vi "SVI_SendSerialCommand.vi"(8 "error in (no error)":errorcluster, 9 "DAC Voltage (mV)":i32, 10 "Address":string="1202", 11 "VISA Refnum in":refnum<visa-resource-name>) -> (0 "error out":errorcluster, 2 "String":string, 3 "VISA Refnum out":refnum<visa-resource-name>)   [LabVIEW 2014]
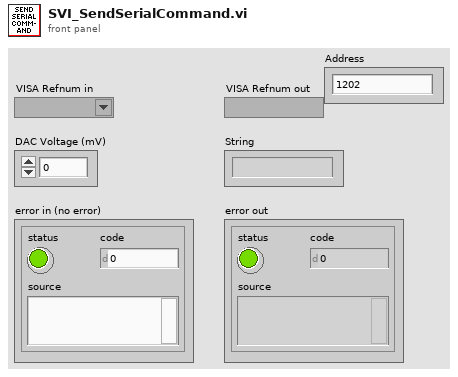
[diagram p1: front panel]
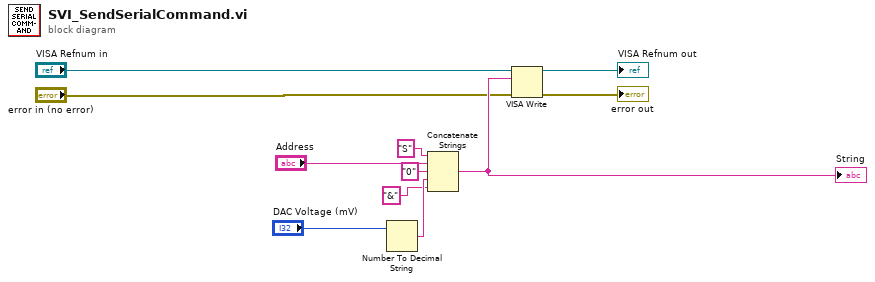
[diagram p0: block diagram]
diagram:
  n1 = Number To Decimal String(number="DAC Voltage (mV)") -> (decimal integer string=w2:string)  [unwired: 1 in]
  n2 = Concatenate Strings("S" ("string"), "Address", "0" ("string"), w2, "&" ("string")) -> (w10:string)
  "String" <- w10
  n3 = VISA Write(VISA resource name="VISA Refnum in", write buffer=w10, error in (no error)="error in (no error)") -> (VISA resource name out=→"VISA Refnum out":refnum<visa-resource-name>, error out=→"error out":errorcluster)  [unwired: 1 out]
